vi "motorMove-Old-Controllers.vi"(3 "Motor (XYZ)":string(combo)="X", 4 "position":dbl, 5 "Device in":refnum<k24>) -> (2 "Device out":refnum<k24>)   [LabVIEW 2014]
doc: "André Romero - 2017\nandretec@ifsc.usp.br"
uses:
  C:/UserLabs/Andre/LabView2014-32bits/kinesisTec/Kinesis/Thorlabs.MotionControl.TCube.DCServoCLI.dll
  Kinesis/Thorlabs.MotionControl.TCube.DCServoCLI.dll
  motorsGlobalVar.vi
  motor-XYZ-GlobalVar.vi
panel:
  out "timeout i":i32
  out "Delay time":u32
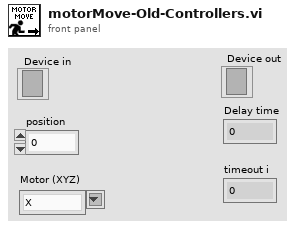
[diagram p1: front panel]
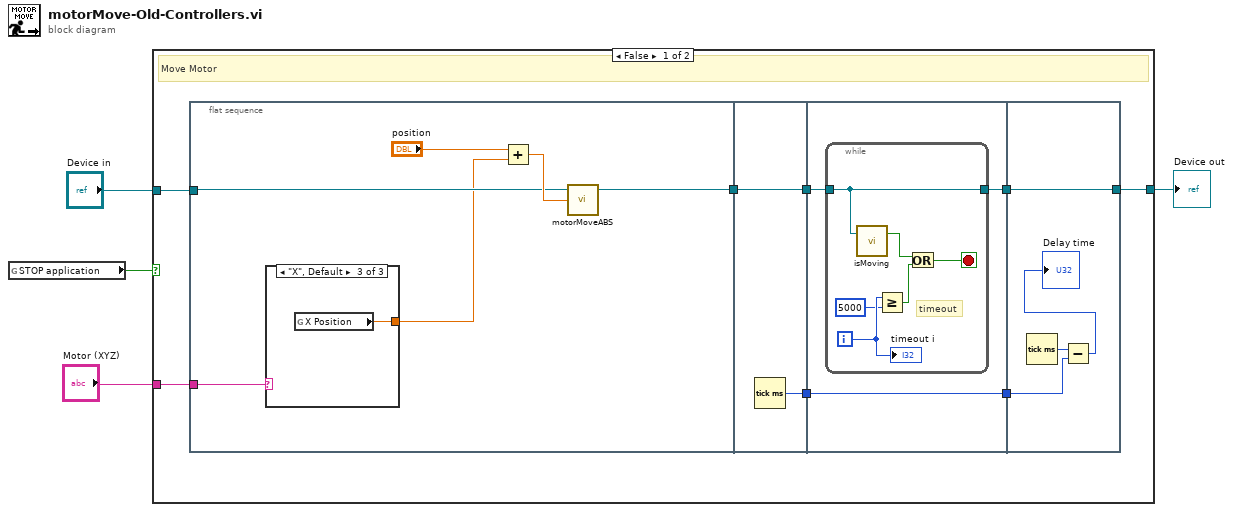
[diagram p0: block diagram]
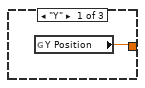
[diagram p2: hidden frame]
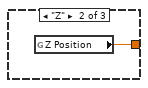
[diagram p3: hidden frame]
diagram:
  n1 = global read "motorsGlobalVar.vi" "STOP application"() -> (w2:bool)
  n2 = case shown="False" w2 {
    tunnel: [w7 w37] -> w4
    tunnel: "Device in" -> [w6 w37]
    tunnel: "Motor (XYZ)" -> [w5 _]
    frame False {
      # "Move Motor"
      n3 = flat-sequence {
        tunnel: [w16] -> w12
        tunnel: w6 -> [w15]
        tunnel: w5 -> [w14]
        tunnel: w12 -> [w23]
        tunnel: [w23] -> w11
        tunnel: [w22] -> w10
        tunnel: w11 -> [w25]
        tunnel: [w26] -> w9
        tunnel: w10 -> [w24]
        tunnel: [w24] -> w8
        tunnel: [w36] -> w7
        tunnel: w9 -> [w36]
        tunnel: w8 -> [w34]
        frame #0 {
          n4 = case shown="\"X\", Default" w14 {
            tunnel: [w19 w20 w21] -> w13
            frame "Y" {
              n5 = global read "motor-XYZ-GlobalVar.vi" "Y Position"() -> (w19:dbl)
            }
            frame "Z" {
              n6 = global read "motor-XYZ-GlobalVar.vi" "Z Position"() -> (w20:dbl)
            }
            frame "X", Default {
              n7 = global read "motor-XYZ-GlobalVar.vi" "X Position"() -> (w21:dbl)
            }
          }
          n8 = Add(x="position", y=w13) -> (x+y=w17:dbl)
          n9 = call "motorMoveABS.vi"("position"=w17, "Device in"=w15) -> ("Device out"=w16:refnum<k24>)  [unwired: 3 in]
        }
        frame #1 {
          n10 = Tick Count (ms)() -> (millisecond timer value=w22:u32)
        }
        frame #2 {
          n11 = while {
            tunnel: [w32] -> w26
            tunnel: w25 -> [w32]
            i -> [w30]
            stop <- w28 stop-if-true
            # "timeout"
            n12 = call "isMoving.vi"("Device in"=w32) -> ("IsMoving"=w31:bool)  [unwired: 2 in]
            n13 = Greater Or Equal?(x=w30, y=5000) -> (x >= y?=w27:bool)
            n14 = Or(x=w31, y=w27) -> (x .or. y?=w28:bool)
            "timeout i" <- w30
          }
        }
        frame #3 {
          n15 = Tick Count (ms)() -> (millisecond timer value=w35:u32)
          n16 = Subtract(x=w35, y=w34) -> (x-y=→"Delay time":u32)
        }
      }
    }
    frame True {
      # "if STOP is TRUE -> stop application"
    }
  }
  "Device out" <- w4
